vi "c_Read Header.vi"() -> (1 "Case Label":T1="Read Header")   [LabVIEW 2020, in "TCP Receive.lvclass"]
uses:
  TCP Receive.lvclass
  <vilib>/addons/_Workers/Library/Case Label.ctl
  <vilib>/addons/_Workers/Library/Workers.lvlib
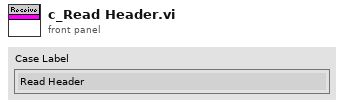
[diagram p1: front panel]
types:
  T1 = typedef "Workers.lvlib/Case Label.ctl" = string
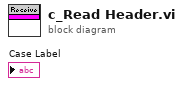
[diagram p0: block diagram]
diagram:
